vi "Destroy.vi"(8 "error in (no error)":errorcluster, 11 "Event Registration Refnum":refnum<event-registration>) -> (0 "error out":errorcluster)   [LabVIEW 2020, in "WebServiceImporter.lvlib" / "Main Panel.lvlib" / "Select Methods.lvlib" / "Events.lvlib"]
uses:
  <vilib>/Platform/WebService/Main Panel/Pages/Select Methods/Events/Events.lvlib
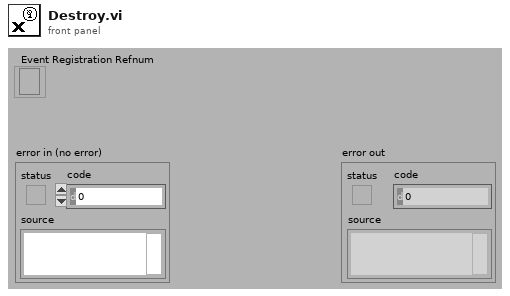
[diagram p1: front panel]
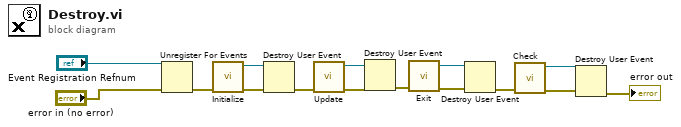
[diagram p0: block diagram]
diagram:
  n1 = Unregister For Events(event registration refnum="Event Registration Refnum", error in="error in (no error)") -> (error out=w9:errorcluster)
  n2 = call <vilib>:"Initialize.vi"("error in (no error)"=w9) -> ("error out"=w10:errorcluster, "user event (out)"=w14:refnum<user-event>)  [unwired: 9 in]
  n3 = Destroy User Event(user event=w14, error in=w10) -> (error out=w8:errorcluster)
  n4 = call <vilib>:"Update.vi"("error in (no error)"=w8) -> ("error out"=w6:errorcluster, "user event (out)"=w7:refnum<user-event>)  [unwired: 9 in]
  n5 = Destroy User Event(user event=w7, error in=w6) -> (error out=w5:errorcluster)
  n6 = call <vilib>:"Exit.vi"("error in (no error)"=w5) -> ("error out"=w4:errorcluster, "user event (out)"=w13:refnum<user-event>)  [unwired: 9 in]
  n7 = Destroy User Event(user event=w13, error in=w4) -> (error out=w1:errorcluster)
  n8 = call <vilib>:"Check.vi"("error in (no error)"=w1) -> ("error out"=w2:errorcluster, "user event (out)"=w3:refnum<user-event>)  [unwired: 9 in]
  n9 = Destroy User Event(user event=w3, error in=w2) -> (error out=→"error out":errorcluster)
